vi "4Pi Dual DM - Active Mirror AE.vi"(2 "Action":T1, 7 "Active Mirror In":i32) -> (8 "Active Mirror":i32)   [LabVIEW 2016]
uses:
  4Pi Dual DM - Controls/4Pi Dual DM - Standard Action.ctl
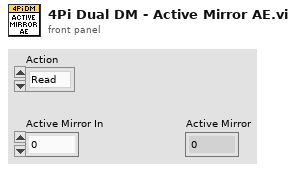
[diagram p1: front panel]
types:
  T1 = typedef "4Pi Dual DM - Standard Action.ctl" = enum16{"Read", "Write"}
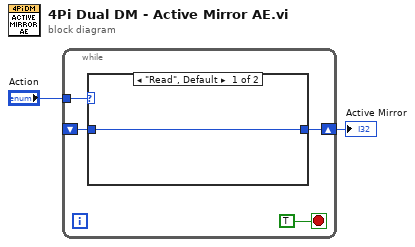
[diagram p0: block diagram]
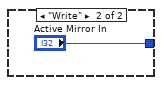
[diagram p2: hidden frame]
diagram:
  n1 = while {
    shift-right: [w4] -> w1
    shift-left: _ -> [w3]
    tunnel: "Action" -> [w5]
    stop <- TRUE stop-if-true
    n2 = case shown="\"Read\", Default" w5 {
      tunnel: [w7 "Active Mirror In"] -> w4
      tunnel: w3 -> [w7 _]
      frame "Read", Default {
      }
      frame "Write" {
      }
    }
  }
  "Active Mirror" <- w1
